vi "Configure Channel (mA Sqrt).vi"(0 "VISA resource name":refnum<visa-resource-name>, 1 "Scaling":T3={"Floating point position (2)"=2, "Lower Scaling (0.0)"=0.0, "Upper Scaling (100.0)"=100.0, "Unit Character (\"\")"=""} {"Upper Scaling (100.0)" format="%_6g"; "Lower Scaling (0.0)" format="%_6g"; "Floating point position (2)" min=0 max=5 step=1}, 2 "Low cut":T2 {"Output (0: Zero)" items=["Zero", "Linear"]; "Low-cut (0.0)" min=0.0 max=5.0 step=0.1 format="%.1g"}, 5 "Channel (0001)":string="0001", 7 "Enable Channel (True)":bool=TRUE, 9 "Range And Span":T1={"mA Range (0 : 0-20mA)"=0, "Enable Span (False)"=FALSE, "Lower Span (0.000)"=0.0, "Upper Span (20.000)"=20.0, "Bias (0)"=0.0} {"mA Range (0 : 0-20mA)" items=["0-20mA"]; "Bias (0)" format="%_6g"; "Upper Span (20.000)" step=0.001 format="%.3g"; "Lower Span (0.000)" step=0.001 format="%.3g"}, 11 "error in (no error)":errorcluster) -> (4 "VISA resource name out":refnum<visa-resource-name>, 6 "Channel":string, 15 "error out":errorcluster)   [LabVIEW 2020, in "Yokogawa GX Series.lvlib"]
doc: "Sets the input range as voltage.\n\nCommand: SRangeAI"
uses:
  <instrlib>/Yokogawa GX Series/Yokogawa GX Series.lvlib
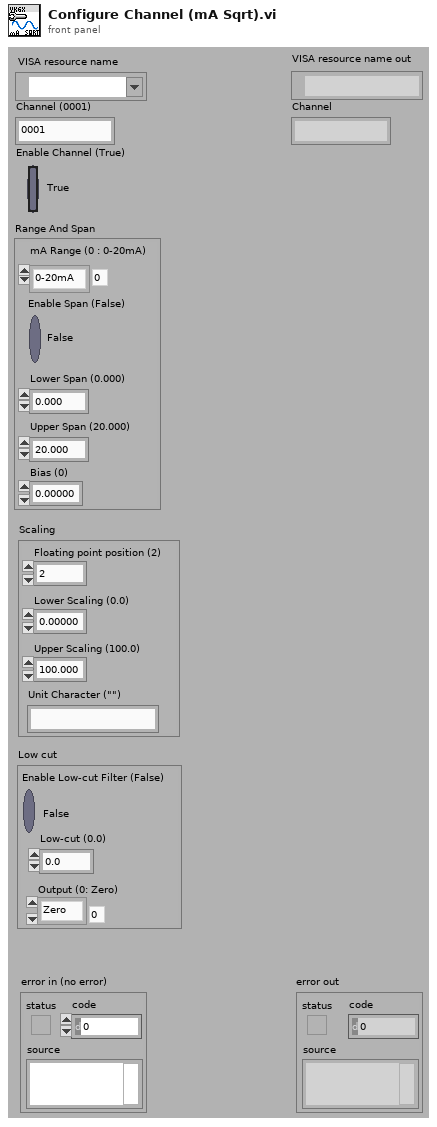
[diagram p1: front panel]
types:
  T1 = cluster{"mA Range (0 : 0-20mA)":i32, "Enable Span (False)":bool, "Lower Span (0.000)":dbl, "Upper Span (20.000)":dbl, "Bias (0)":dbl}
  T2 = cluster{"Enable Low-cut Filter (False)":bool, "Low-cut (0.0)":dbl, "Output (0: Zero)":u16}
  T3 = cluster{"Floating point position (2)":i32, "Lower Scaling (0.0)":dbl, "Upper Scaling (100.0)":dbl, "Unit Character (\"\")":string}
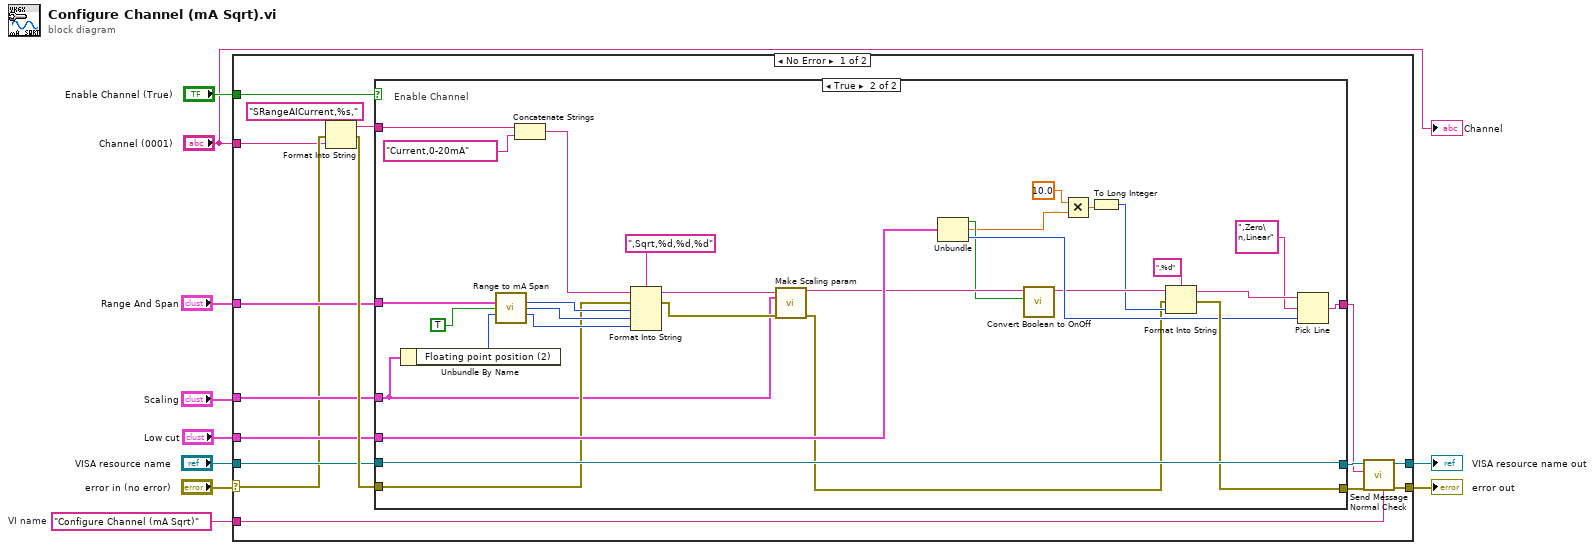
[diagram p0: block diagram]
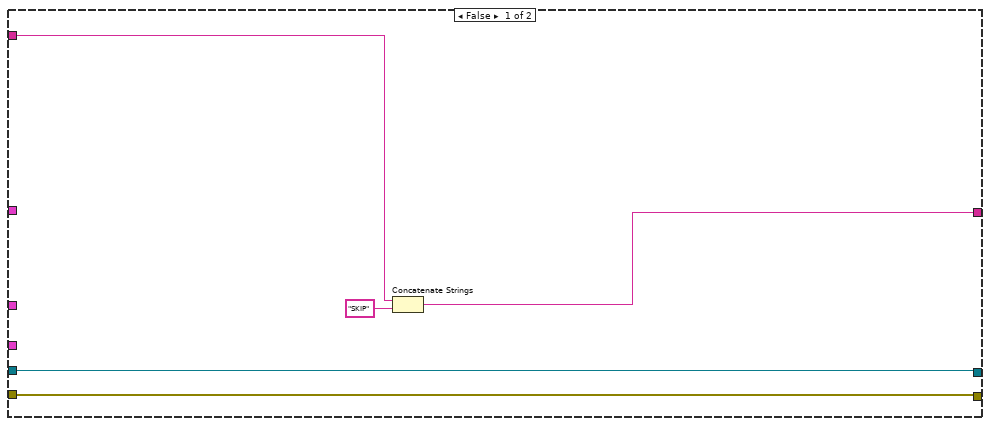
[diagram p2: hidden frame]
diagram:
  w4 = "Configure Channel (mA Sqrt)"  # VI name
  n1 = case shown="No Error" "error in (no error)" {
    selector: "error in (no error)" -> [w16 w62]
    tunnel: "Enable Channel (True)" -> [w15 _]
    tunnel: "VISA resource name" -> [w23 w63]
    tunnel: "Scaling" -> [w22 _]
    tunnel: "Low cut" -> [w21 _]
    tunnel: [w11 w63] -> w6
    tunnel: [w12 w62] -> w5
    tunnel: w4 -> [w18 _]
    tunnel: "Range And Span" -> [w17 _]
    tunnel: "Channel (0001)" -> [w14 _]
    frame No Error {
      n2 = Format Into String(format string="SRangeAICurrent,%s,", error in=w16, w14) -> (resulting string=w24:string, error out=w25:errorcluster)  [unwired: 1 in]
      n3 = case shown="True" w15 {
        tunnel: w25 -> [w28 w55]
        tunnel: [w28 w54] -> w13
        tunnel: w24 -> [w29 w51]
        tunnel: [w31 w47] -> w19
        tunnel: w23 -> [w27 w56]
        tunnel: [w27 w56] -> w20
        tunnel: w17 -> [_ w35]
        tunnel: w22 -> [_ w38]
        tunnel: w21 -> [_ w57]
        frame False {
          n4 = Concatenate Strings(w29, "SKIP") -> (w31:string)
        }
        frame True {
          # "Enable Channel"
          n5 = Unbundle By Name(w38) -> ("Floating point position (2)"=w43:i32)
          n6 = call <instrlib>:"Range to mA Span.vi"("Span"=w35, "Scaling? (False)"=TRUE, "Floating Point Position (2)"=w43) -> ("Lower Span"=w60:i32, "Upper Span"=w59:i32, "Bias"=w58:i32)  [unwired: 10 in]
          n7 = Concatenate Strings(w51, "Current,0-20mA") -> (w34:string)
          n8 = Format Into String(format string=",Sqrt,%d,%d,%d", initial string=w34, error in=w55, w60, w59, w58) -> (resulting string=w39:string, error out=w41:errorcluster)
          n9 = call <instrlib>:"Make Scaling param.vi"("String (\"\")"=w39, "Scaling"=w38, "error in (no error)"=w41) -> ("String After"=w37:string, "error out"=w40:errorcluster)  [unwired: 11 in]
          n10 = Unbundle(w57) -> ("Enable Low-cut Filter (False)"=w33:bool, "Low-cut (0.0)"=w32:dbl, "Output (0: Zero)"=w52:u16)
          n11 = call <instrlib>:"Convert Boolean to OnOff.vi"("On/Off"=w33, "Initial String (\"\")"=w37) -> ("Resulting String"=w50:string)  [unwired: 9 in]
          n12 = Multiply(x=10.0, y=w32) -> (x*y=w45:dbl)
          n13 = To Long Integer(number=w45) -> (32bit integer=w44:i32)
          n14 = Format Into String(format string=",%d", initial string=w50, error in=w40, w44) -> (resulting string=w49:string, error out=w54:errorcluster)
          n15 = Pick Line(string ("")=w49, multi-line string=",Zero\n,Linear", line index=w52) -> (output string=w47:string)
        }
      }
      n16 = call <instrlib>:"Send Message Normal Check.vi"("Source (\"\")"=w18, "error in (no error)"=w13, "Send Message (\"\")"=w19, "VISA resource name"=w20) -> ("error out"=w12:errorcluster, "VISA resource name out"=w11:refnum<visa-resource-name>)  [unwired: 2 in, 4 out]
    }
    frame Error {
    }
  }
  "error out" <- w5
  "VISA resource name out" <- w6
  "Channel" <- "Channel (0001)"
